vi "ConfigureCamera.vi"(8 "error in (no error)":errorcluster, 11 "Refnum in":T1) -> (0 "error out":errorcluster, 3 "Refnum out":T1)   [LabVIEW 2015]
uses:
  <vilib>/userdefined/High Color/IMAQdx.ctl
  <resource>/objmgr/imaqdx.rc
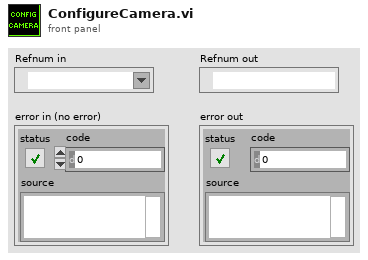
[diagram p1: front panel]
types:
  T1 = typedef "IMAQdx.ctl" = refnum<k21>
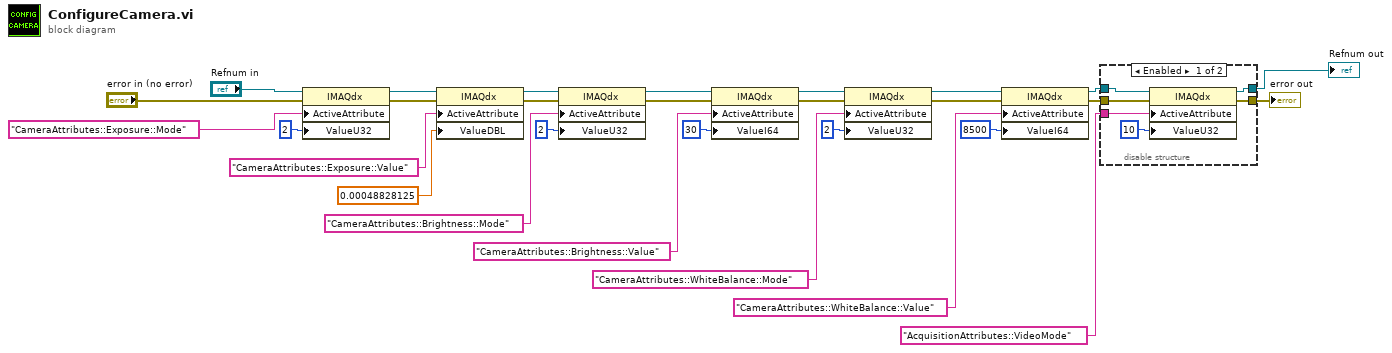
[diagram p0: block diagram]
diagram:
  n1 = property class="IMAQdx"(reference="Refnum in", error in="error in (no error)", "ActiveAttribute"="CameraAttributes::Exposure::Mode", "ValueU32"=u32 2) -> (reference out=w5:T1, error out=w6:errorcluster)
  n2 = property class="IMAQdx"(reference=w5, error in=w6, "ActiveAttribute"="CameraAttributes::Exposure::Value", "ValueDBL"=0.00048828125) -> (reference out=w12:T1, error out=w13:errorcluster)
  n3 = property class="IMAQdx"(reference=w12, error in=w13, "ActiveAttribute"="CameraAttributes::Brightness::Mode", "ValueU32"=u32 2) -> (reference out=w9:T1, error out=w10:errorcluster)
  n4 = property class="IMAQdx"(reference=w9, error in=w10, "ActiveAttribute"="CameraAttributes::Brightness::Value", "ValueI64"=i64 30) -> (reference out=w18:T1, error out=w19:errorcluster)
  n5 = property class="IMAQdx"(reference=w18, error in=w19, "ActiveAttribute"="CameraAttributes::WhiteBalance::Mode", "ValueU32"=u32 2) -> (reference out=w16:T1, error out=w17:errorcluster)
  n6 = property class="IMAQdx"(reference=w16, error in=w17, "ActiveAttribute"="CameraAttributes::WhiteBalance::Value", "ValueI64"=i64 8500) -> (reference out=w24:T1, error out=w25:errorcluster)
  n7 = disable-structure shown="Enabled" {
    disable-tunnel: [w35 w36] -> w29
    disable-tunnel: [w34 w37] -> w28
    disable-tunnel: w25 -> [w32 w36]
    disable-tunnel: w24 -> [w31 w37]
    disable-tunnel: "AcquisitionAttributes::VideoMode" ("ActiveAttribute") -> [w30 _]
    frame Enabled {
      n8 = property class="IMAQdx"(reference=w31, error in=w32, "ActiveAttribute"=w30, "ValueU32"=u32 10) -> (reference out=w34:T1, error out=w35:errorcluster)
    }
    frame Disabled {
    }
  }
  "error out" <- w29
  "Refnum out" <- w28
